vi "ICE450 Ultra Initialization.vi"(8 "error in (no error)":errorcluster, 10 "delay before read (ms)":u32=500, 11 "VISA resource name":refnum<visa-resource-name>) -> (2 "Repetition rate":dbl, 3 "Laser initialization status":string)   [LabVIEW 2016]
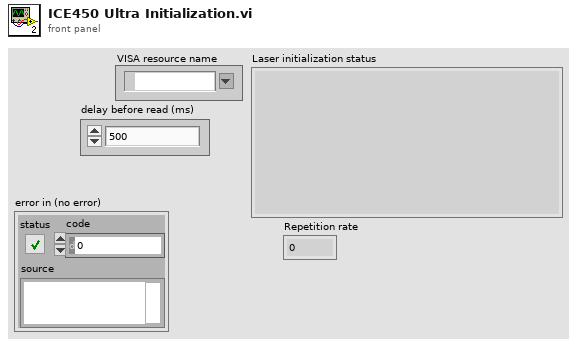
[diagram p1: front panel]
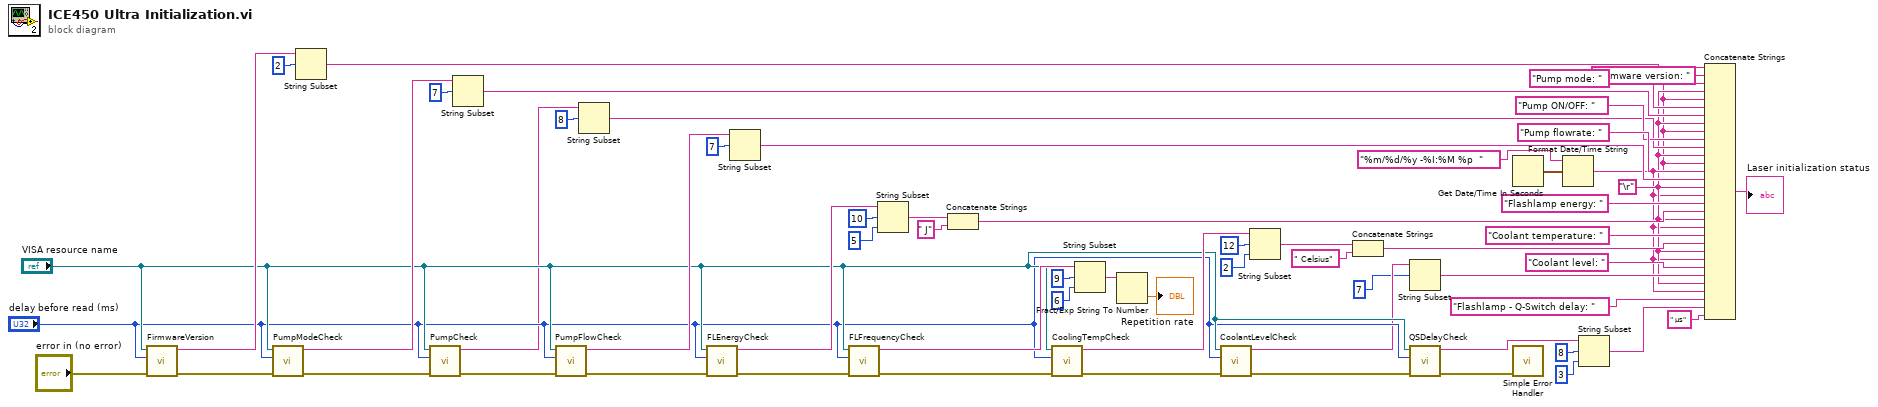
[diagram p0: block diagram]
diagram:
  w8 = "\r"
  n1 = call "FirmwareVersion.vi"("Error In"="error in (no error)", "delay before read (ms)"="delay before read (ms)", "VISA resource name"="VISA resource name") -> ("Error Out"=w26:errorcluster, "read buffer"=w41:string)  [unwired: 5 in, 2 out]
  n2 = call "PumpModeCheck.vi"("Error In"=w26, "delay before read (ms)"="delay before read (ms)", "VISA resource name"="VISA resource name") -> ("Error Out"=w27:errorcluster, "read buffer"=w43:string)  [unwired: 5 in, 2 out]
  n3 = String Subset(string=w41, offset (0)=2) -> (substring=w47:string)  [unwired: 1 in]
  n4 = call "PumpCheck.vi"("Error In"=w27, "delay before read (ms)"="delay before read (ms)", "VISA resource name"="VISA resource name") -> ("Error Out"=w25:errorcluster, "read buffer"=w13:string)  [unwired: 5 in, 2 out]
  n5 = String Subset(string=w43, offset (0)=7) -> (substring=w45:string)  [unwired: 1 in]
  n6 = call "PumpFlowCheck.vi"("Error In"=w25, "delay before read (ms)"="delay before read (ms)", "VISA resource name"="VISA resource name") -> ("Error Out"=w24:errorcluster, "read buffer"=w50:string)  [unwired: 5 in, 2 out]
  n7 = String Subset(string=w13, offset (0)=8) -> (substring=w12:string)  [unwired: 1 in]
  n8 = call "FLEnergyCheck.vi"("Error In"=w24, "delay before read (ms)"="delay before read (ms)", "VISA resource name"="VISA resource name") -> ("Error Out"=w23:errorcluster, "read buffer"=w20:string)  [unwired: 5 in, 2 out]
  n9 = String Subset(string=w50, offset (0)=7) -> (substring=w51:string)  [unwired: 1 in]
  n10 = call "FLFrequencyCheck.vi"("Error In"=w23, "delay before read (ms)"="delay before read (ms)", "VISA resource name"="VISA resource name") -> ("Error Out"=w22:errorcluster, "read buffer"=w33:string)  [unwired: 5 in, 2 out]
  n11 = String Subset(string=w20, offset (0)=10, length (rest)=5 ("length (rest)")) -> (substring=w52:string)
  n12 = Concatenate Strings(w52, " J" ("string")) -> (w55:string)
  n13 = call "CoolingTempCheck.vi"("Error In"=w22, "delay before read (ms)"="delay before read (ms)", "VISA resource name"="VISA resource name") -> ("Error Out"=w21:errorcluster, "read buffer"=w59:string)  [unwired: 5 in, 2 out]
  n14 = String Subset(string=w33, offset (0)=9, length (rest)=6 ("length (rest)")) -> (substring=w34:string)
  n15 = Fract/Exp String To Number(string=w34) -> (number=→"Repetition rate":dbl)  [unwired: 3 in, 1 out]
  n16 = call "CoolantLevelCheck.vi"("Error In"=w21, "delay before read (ms)"="delay before read (ms)", "VISA resource name"="VISA resource name") -> ("Error Out"=w35:errorcluster, "read buffer"=w10:string)  [unwired: 5 in, 2 out]
  n17 = String Subset(string=w59, offset (0)=12, length (rest)=2 ("length (rest)")) -> (substring=w60:string)
  n18 = Concatenate Strings(w60, " Celsius" ("string")) -> (w62:string)
  n19 = String Subset(string=w10, offset (0)=7) -> (substring=w9:string)  [unwired: 1 in]
  n20 = call "QSDelayCheck.vi"("Error In"=w35, "delay before read (ms)"="delay before read (ms)", "VISA resource name"="VISA resource name") -> ("Error Out"=w39:errorcluster, "read buffer"=w38:string)  [unwired: 5 in, 2 out]
  n21 = Get Date/Time In Seconds() -> (seconds since 1Jan1904=w29:timestamp)
  n22 = call <vilib>:"Simple Error Handler.vi"("error in (no error)"=w39) -> ()  [unwired: 4 in, 5 out]
  n23 = Format Date/Time String(time format string (%c)="%m/%d/%y -%I:%M %p  ", seconds (now)=w29) -> (date/time string=w3:string)  [unwired: 1 in]
  n24 = String Subset(string=w38, offset (0)=8, length (rest)=3 ("length (rest)")) -> (substring=w6:string)
  n25 = Concatenate Strings(w3, "Firmware version: " ("string"), w47, w8, w3, "Pump mode: " ("string"), w45, w8, w3, "Pump ON/OFF: " ("string"), w12, w8, w3, "Pump flowrate: " ("string"), w51, w8, w3, "Flashlamp energy: " ("string"), w55, w8, w3, "Coolant temperature: " ("string"), w62, w8, w3, "Coolant level: " ("string"), w9, w8, w3, "Flashlamp - Q-Switch delay: " ("string"), w6, " µs" ("string")) -> (→"Laser initialization status":string)
